vi "ftrans.vi"(10 "F":dbl[](array[numeric]), 11 "T":T1) -> (2 "Ft":dbl[](array[numeric]))   [LabVIEW 2017, in "NI_Kinematics.lvlib"]
uses:
  <vilib>/robotics/Kinematics/NI_Kinematics.lvlib
  <vilib>/Analysis/Matrix/Datatypes/RealMatrix.ctl
  <vilib>/Analysis/baseanly.llb/A x Vector.vi
  <vilib>/Analysis/NI_AALPro.lvlib
  <vilib>/Analysis/NI_AALBase.lvlib
  <vilib>/Analysis/Matrix/NI_Matrix.lvlib
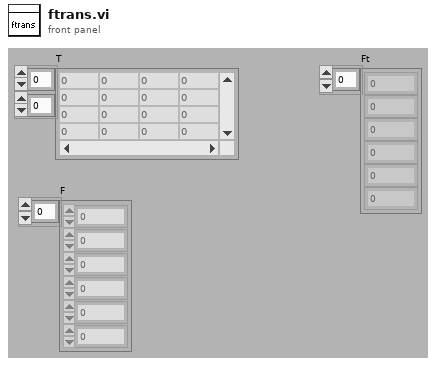
[diagram p1: front panel]
types:
  T1 = typedef "NI_Matrix.lvlib/RealMatrix.ctl" = dbl[][]
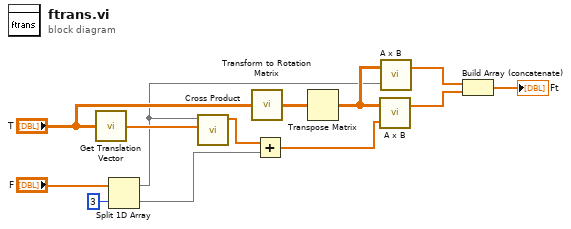
[diagram p0: block diagram]
diagram:
  n1 = call <vilib>:"Get Translation Vector.vi"("transform"="T") -> ("translation vector"=w11:dbl[])
  n2 = Split 1D Array(array="F", index=3) -> (first subarray=w4:dbl[], second subarray=w10:dbl[])
  n3 = call <vilib>:"Cross Product.vi"("B Vector"=w11, "A Vector"=w4) -> ("Cross Product"=w9:dbl[])  [unwired: 8 in, 1 out]
  n4 = call <vilib>:"Transform to Rotation Matrix.vi"("transform"="T") -> ("rotation matrix"=w7:T1)
  n5 = Add(x=w9, y=w10) -> (x+y=w6:dbl[])
  n6 = Transpose Matrix(1:w7) -> (0:w5:T1)
  n7 = call-poly <vilib>:"A x B.vi"("Vector"=w6, "A"=w5) -> ("A x Vector"=w3:dbl[])  [unwired: 1 out]
  n8 = call-poly <vilib>:"A x B.vi"("Vector"=w4, "A"=w5) -> ("A x Vector"=w2:dbl[])  [unwired: 1 out]
  n9 = Build Array (concatenate)(w2, w3) -> (→"Ft":dbl[])
